vi "main.vi"() -> ()   [LabVIEW 2016]
uses:
  <vilib>/Utility/miscctls.llb/LVMajorAndMinorColorsTypeDef.ctl
panel:
  in  "关闭读取刷新？":bool
  out "项名":string[][](array[string])
  out "下位机消息":T1(array[cluster])
  out "输出数组":T2(array[cluster]) {"Data7" format="%x"; "Data6" format="%x"; "Data5" format="%x"; "Data4" format="%x"; "Data3" format="%x"; "Data2" format="%x"; "Data1" format="%x"; "Data0" format="%x"}
  out "发送配置":T3(array[cluster])
  out "OpenDevice":i32
  out "StartCAN_Success":i32
  out "InitCAN_Success":i32
  out "CloseDevice_Success?":u32
  in  "VCI_INIT_CONFIG":T4={"AccCode"=0, "AccMask"=4294967295, "Reserved"=0, "Filter"=0, "Timing0"=0, "Timing1"=28, "Mode"=0} {"AccCode" format="%x"; "AccMask" format="%x"; "Reserved" format="%x"; "Timing1" format="%x"}
  out "项标识符":string
  in  "选项卡控件":enum32{"通用设置", "实时波形", "数据发送", "历史波形"}(tab)
  in  "远程帧标志：":u8
  in  "上传ID":u32=270 format="%x"
  out "启动日志":string
  in  "输出配置路径":path=path "C:/Users/Azmat/Desktop/canTools_v1.0.0/Confs/Send/发送协议.txt"
  in  "掩码：":u32=4294967295 format="%x"
  in  "校验码：":u32 format="%x"
  in  "波特率：":enum16{"100k", "250k", "500k"}(ring)=enum."250k"
  in  "内存地址":u32=15360 format="%x"
  in  "标定站地址":u32=1 format="%x"
  in  "输入配置路径":path=path "C:/Users/Azmat/Desktop/canTools_v1.0.0/Confs/Receive/接收协议.txt"
  in  "颜色库":u32[](array[colorbox])=[16731714, 16769743, 4390903, 16746746, 4390806, 9603948, 16744793, 4481339, 5898174, 16860, 16766786, 16729344, 4390770, 5963865, 16752520, 15597823, 16775072, 46792, 16730368, 7115393, 10122379, 7465727, 7663, 9306367, 16722686, 11800064, 15663104, 3949056, 16752873, 11121548, 2031753, 12976056]
  in  "标定ID":u32=269 format="%x"
  in  "设备索引号：":u32
  in  "Timing0":u8
  in  "Timing1":u8=28 format="%x"
  out "系统状态":bool
  in  "保存波形":bool
  out "Waveform Chart":dbl[][](graph)
  in  "Chart legend":T5(array[cluster])
  in  "启动":bool
  in  "保存发送表":bool
  in  "搜索发送表":bool
  in  "上传":bool
  in  "下载":bool
  in  "发送表":i32[](listbox) caption="多列列表框"
  in  "打开TDMS":bool
  out "波形图":waveform(dbl)[](graph)
  in  "波形图图例":T6(array[cluster])
  in  "开始":dbl
  in  "结束":dbl
  in  "输入/拖动":bool
  out "波形数组out":dbl[](array[numeric])
  out "接受协议数组":T7(array[cluster])
  out "VCI_CAN_OBJ":T8
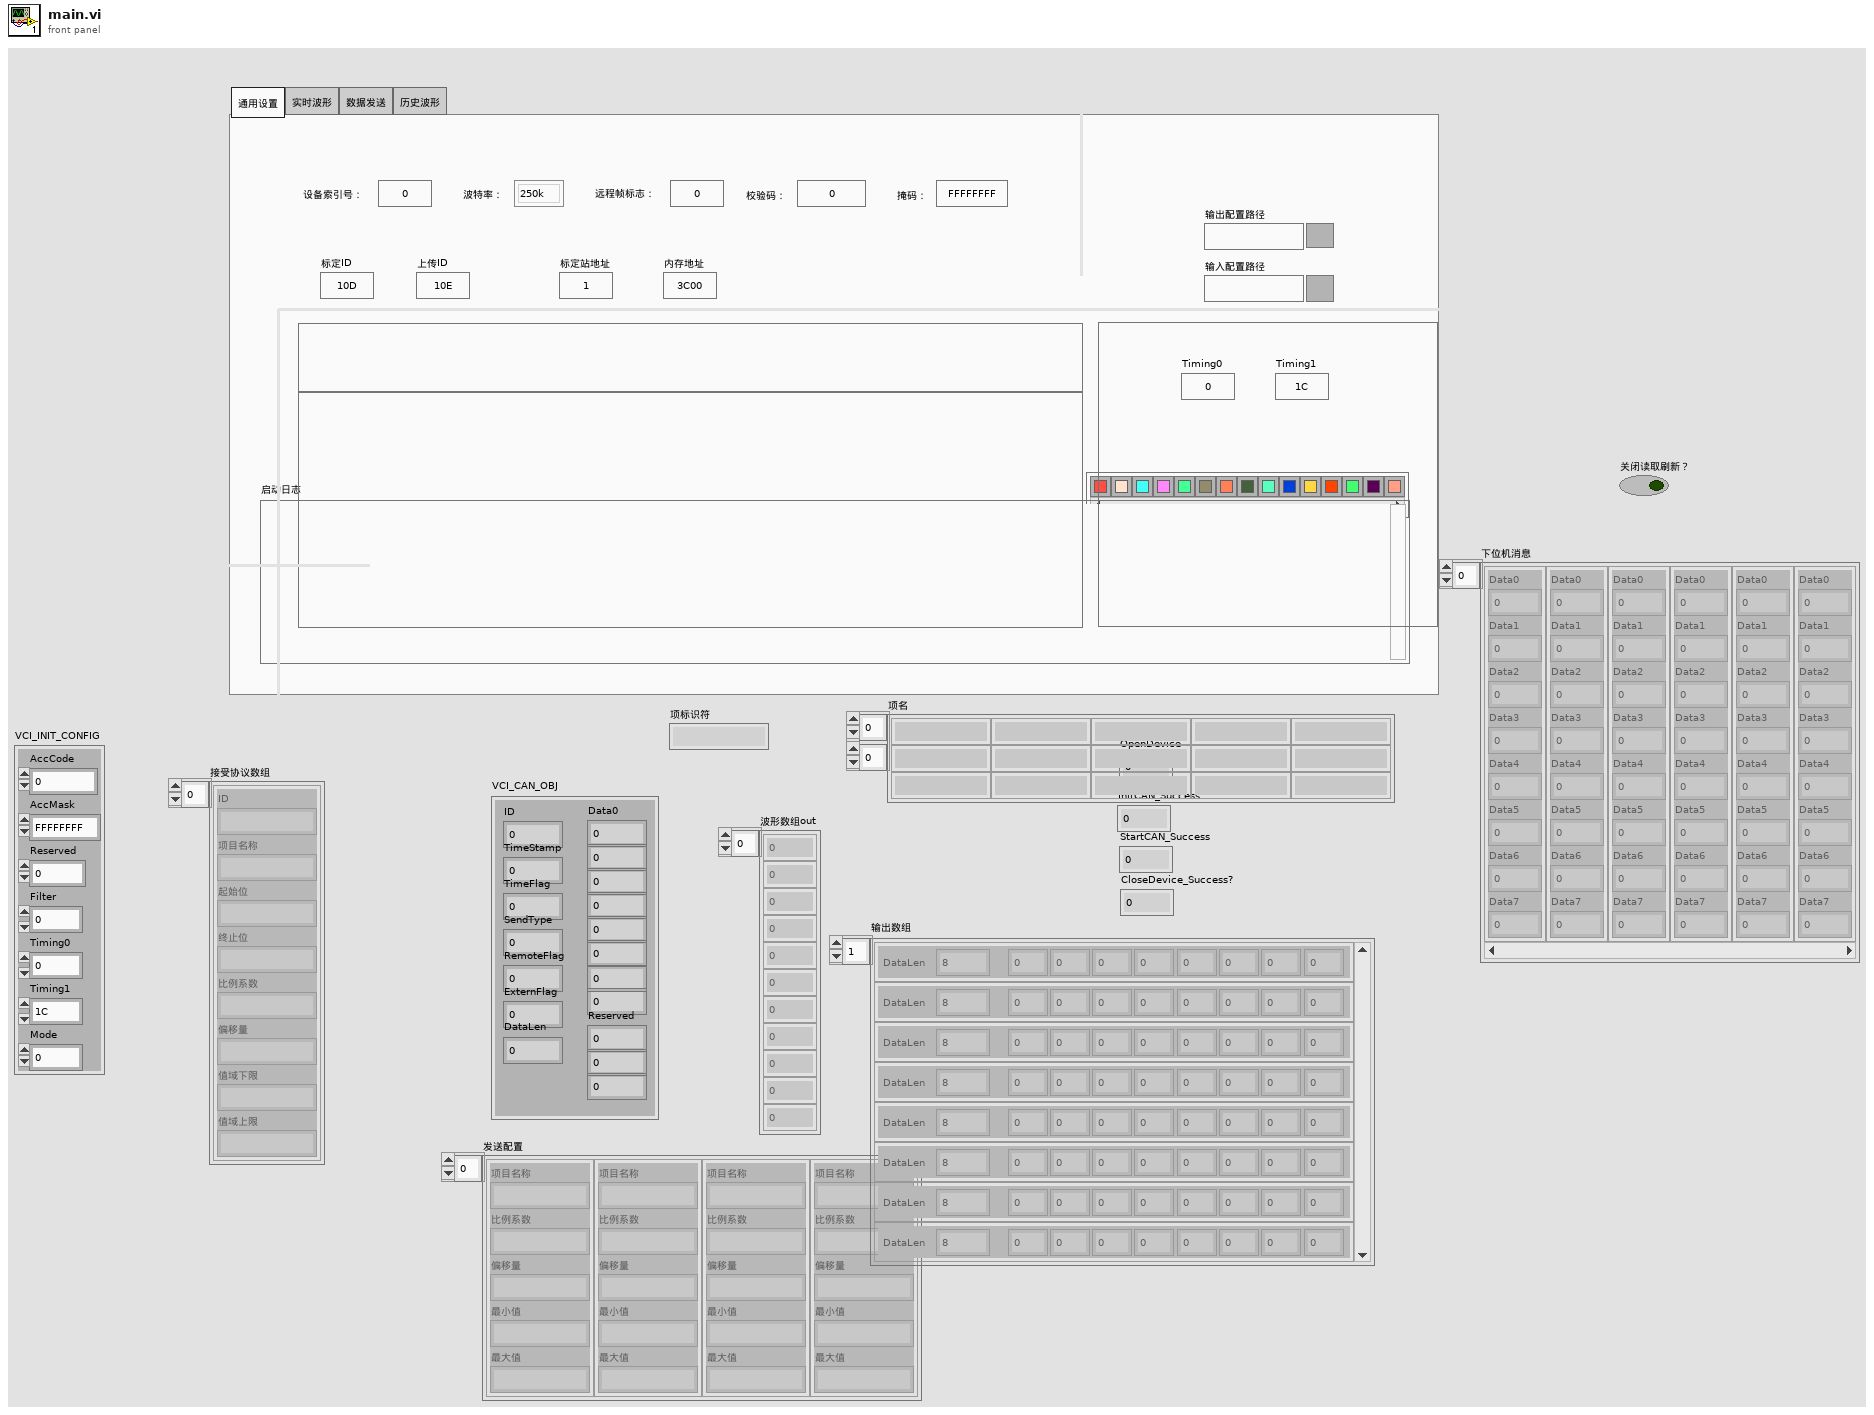
[diagram p1: front panel]
types:
  T1 = cluster{"Data0":u8, "Data1":u8, "Data2":u8, "Data3":u8, "Data4":u8, "Data5":u8, "Data6":u8, "Data7":u8}[]
  T2 = cluster{"Data0":u8, "Data1":u8, "Data2":u8, "Data3":u8, "Data4":u8, "Data5":u8, "Data6":u8, "Data7":u8, "DataLen":u8}[]
  T3 = cluster{"项目名称":string, "比例系数":string, "偏移量":string, "最小值":string, "最大值":string}[]
  T4 = cluster{"AccCode":u32, "AccMask":u32, "Reserved":u32, "Filter":u8, "Timing0":u8, "Timing1":u8, "Mode":u8}
  T5 = cluster{"曲线名称":string, "曲线颜色":u32, "曲线宽度":u16, "当前波形值":dbl, "曲线可见":bool}[]
  T6 = cluster{"曲线名称":string, "曲线颜色":u32, "曲线宽度":u16, "开始":dbl, "曲线可见":bool, "结束":dbl}[]
  T7 = cluster{"ID":string, "项目名称":string, "起始位":string, "终止位":string, "比例系数":string, "偏移量":string, "值域下限":string, "值域上限":string}[]
  T8 = cluster{"ID":u32, "TimeStamp":u32, "TimeFlag":u8, "SendType":i8, "RemoteFlag":u8, "ExternFlag":u8, "DataLen":u8, "Data0":u8, "Data1":u8, "Data2":u8, "Data3":u8, "Data4":u8, "Data5":u8, "Data6":u8, "Data7":u8, "Reserved":u8, u8, u8}
  T9 = cluster{"曲线名称":string, "曲线颜色":u32, "曲线宽度":u16, "当前波形值":dbl, "曲线可见":bool}
  T10 = cluster{"ID":u32, "TimeStamp":u32, "TimeFlag":u8, "SendType":u8, "RemoteFlag":u8, "ExternFlag":u8, "DataLen":u8, "Data0":u8, "data1":u8, "data2":u8, "data3":u8, "data4":u8, "data5":u8, "data6":u8, "data7":u8, "Reserved":u8, u8, u8}
  T11 = enum16{"open", "open or create", "create or replace", "create", "open (read-only)"}
  T12 = cluster{"曲线名称":string, "曲线颜色":u32, "曲线宽度":u16, "开始":dbl, "曲线可见":bool, "结束":dbl}
  T13 = cluster{"data2":u8, "data3":u8, "data4":u8, "data5":u8, "data6":u8, "data7":u8}[]
  T14 = typedef "LVMajorAndMinorColorsTypeDef.ctl" = cluster{"Major Color":u32, "Minor Color":u32}
  T15 = cluster{"曲线名称":string, "曲线颜色":u32, "曲线宽度":u16, "最小值":dbl, "曲线可见":bool, "最大值":dbl}[]
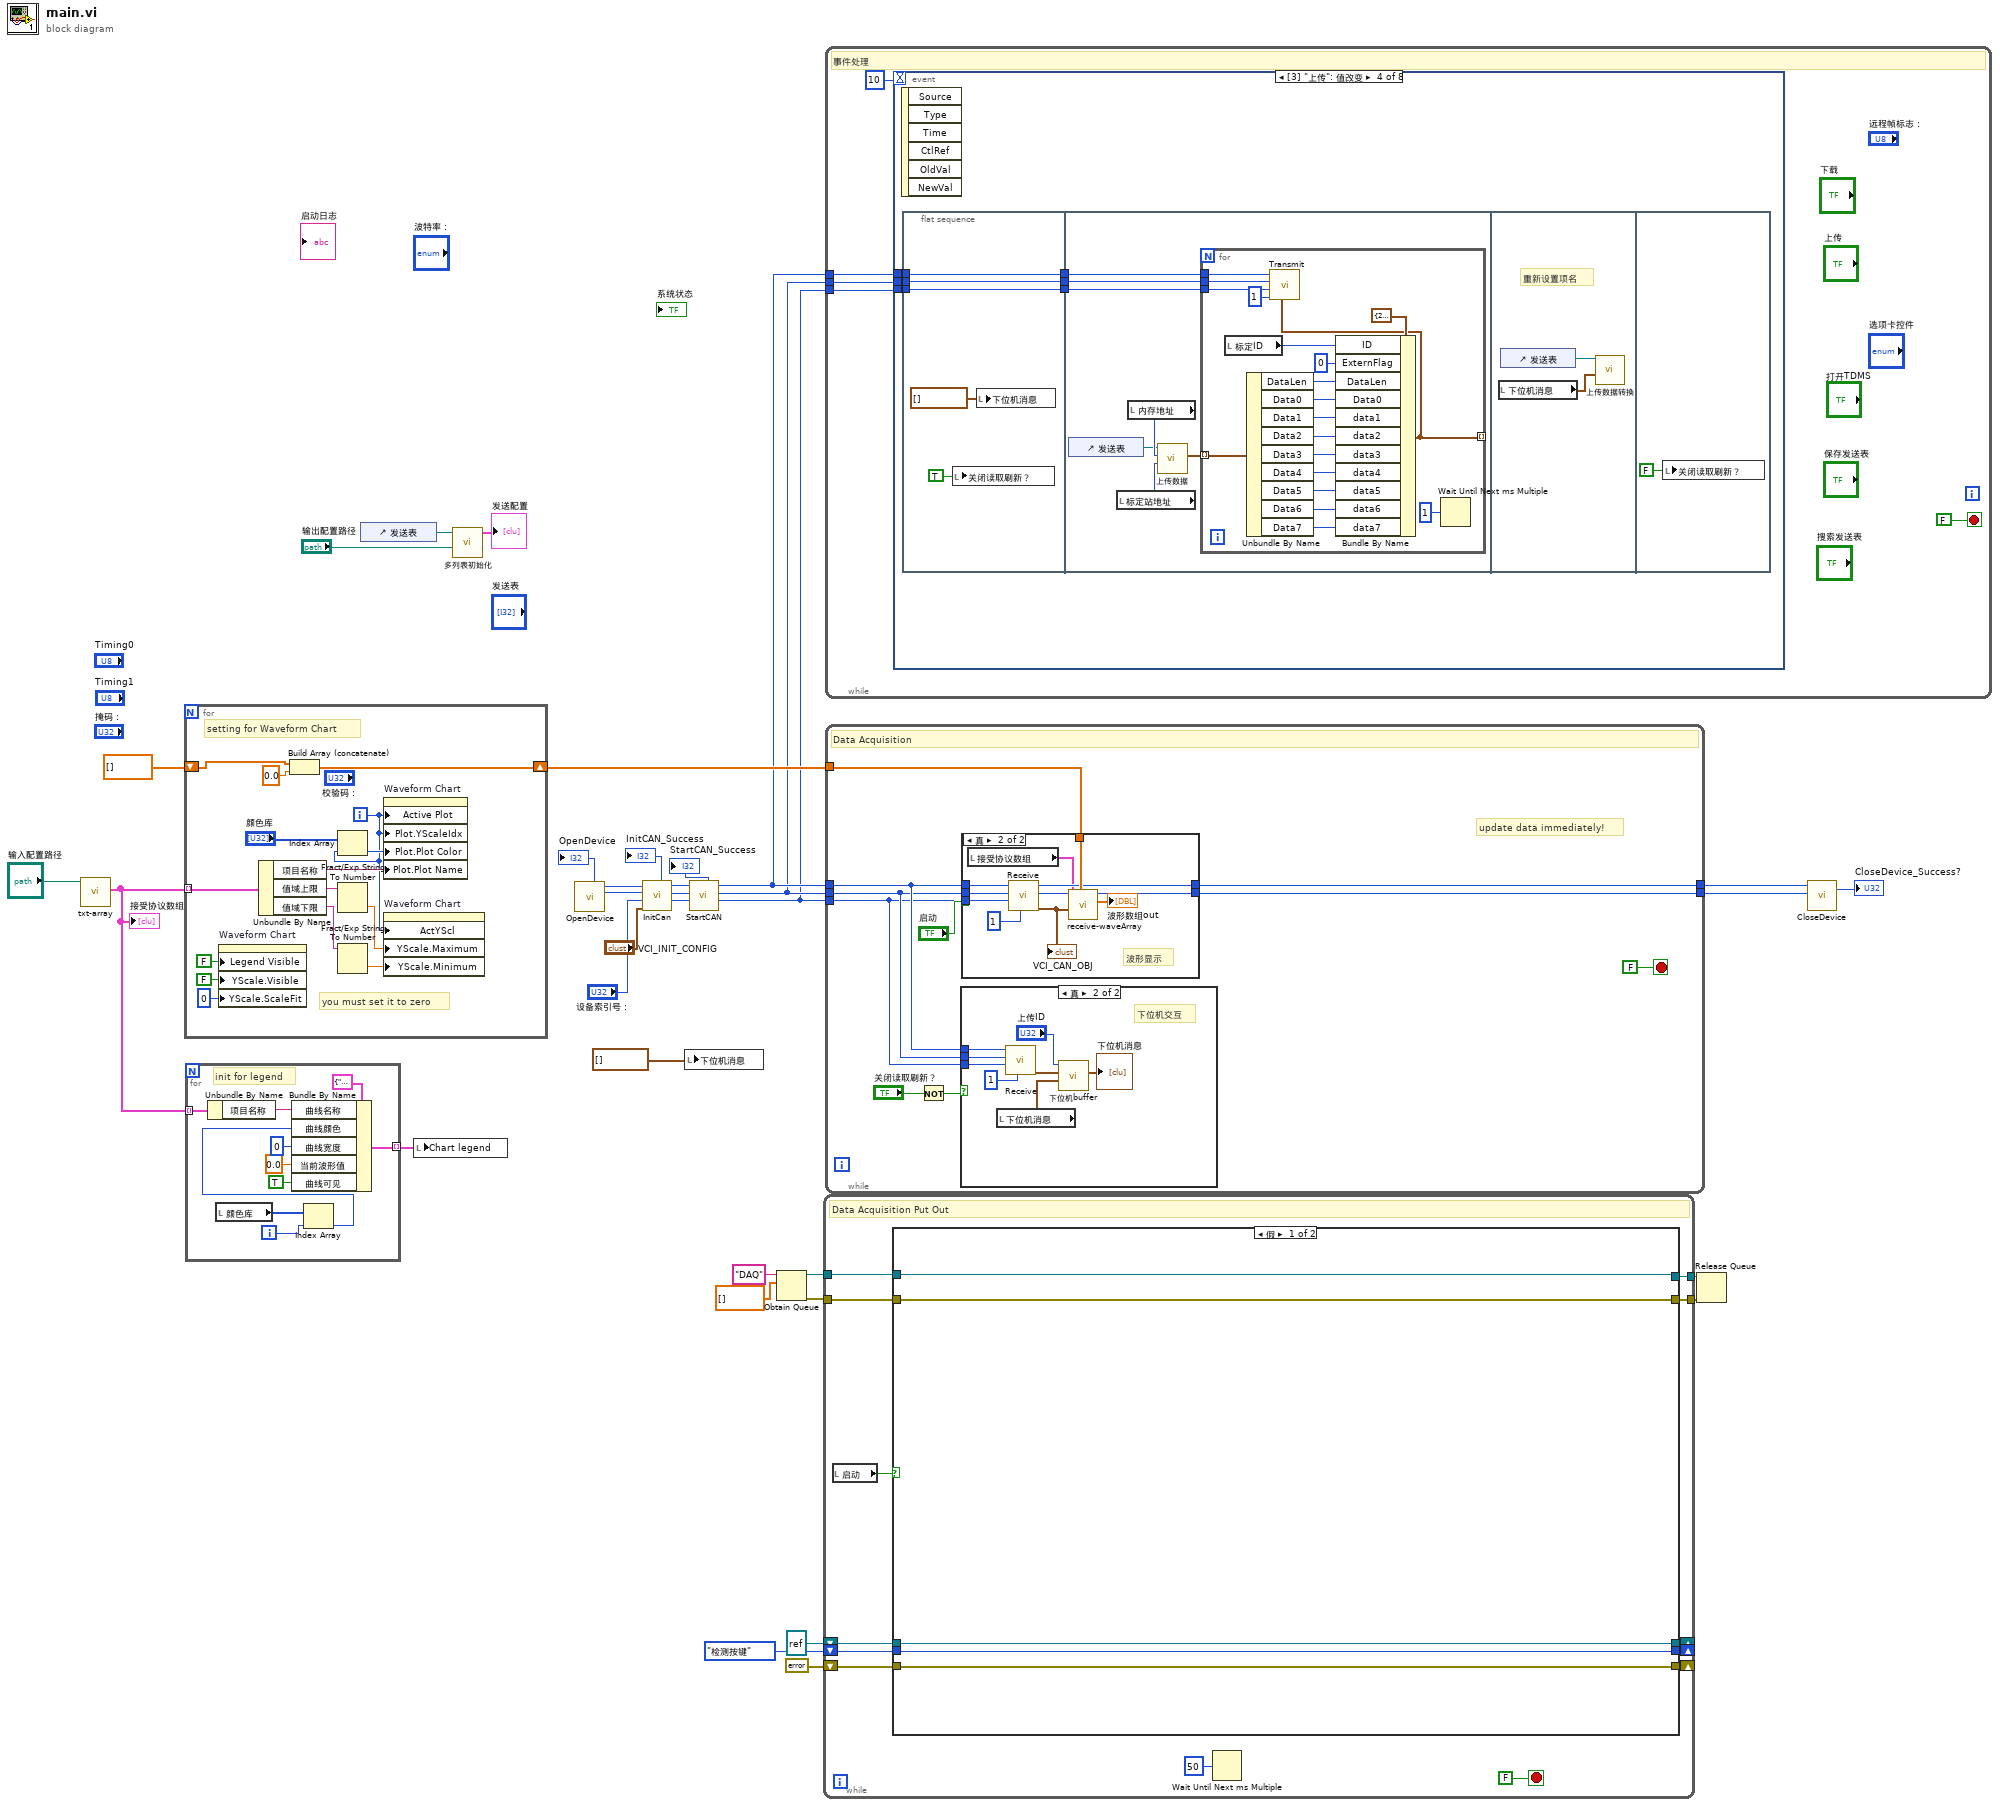
[diagram p0: block diagram]
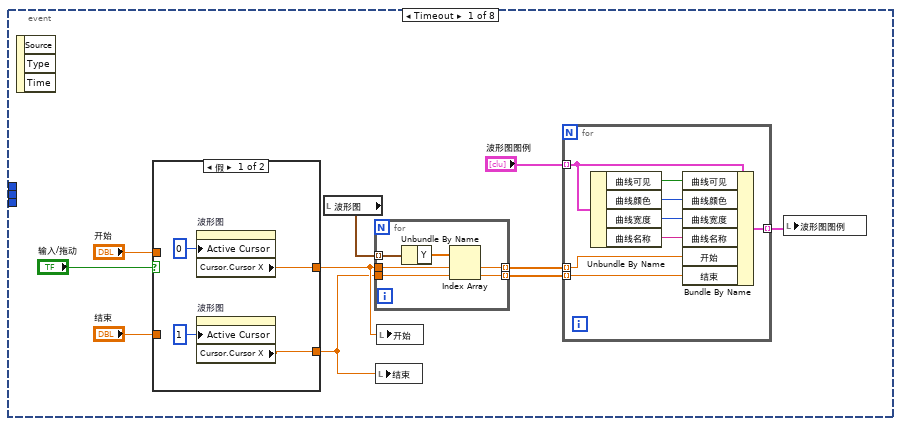
[diagram p2: hidden frame]
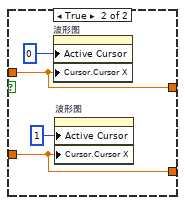
[diagram p3: hidden frame]
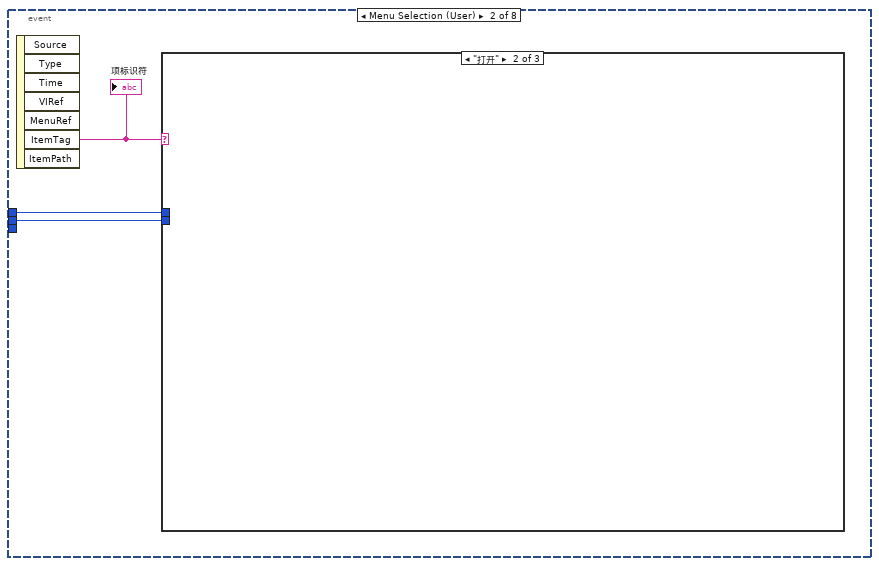
[diagram p4: hidden frame]
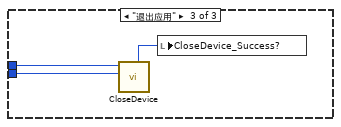
[diagram p6: hidden frame]
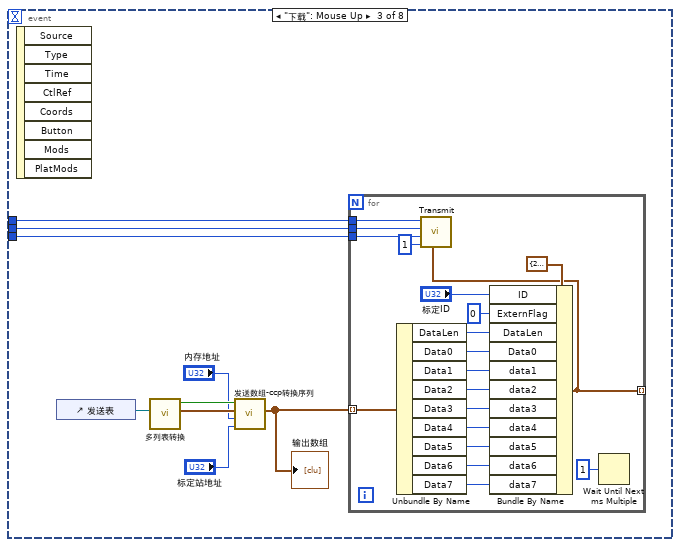
[diagram p7: hidden frame]
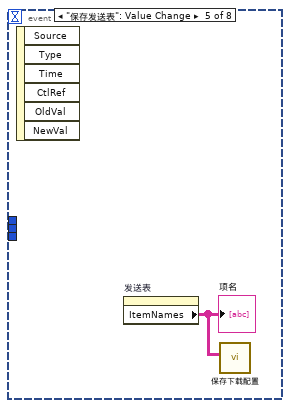
[diagram p8: hidden frame]
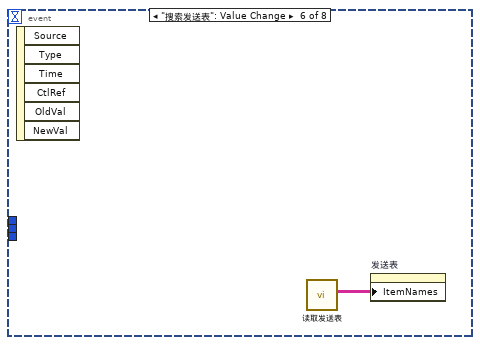
[diagram p9: hidden frame]
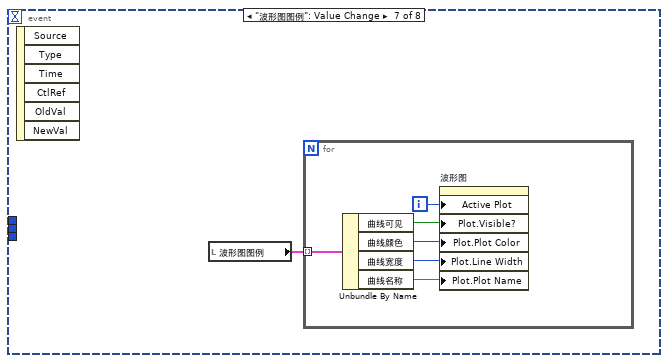
[diagram p10: hidden frame]
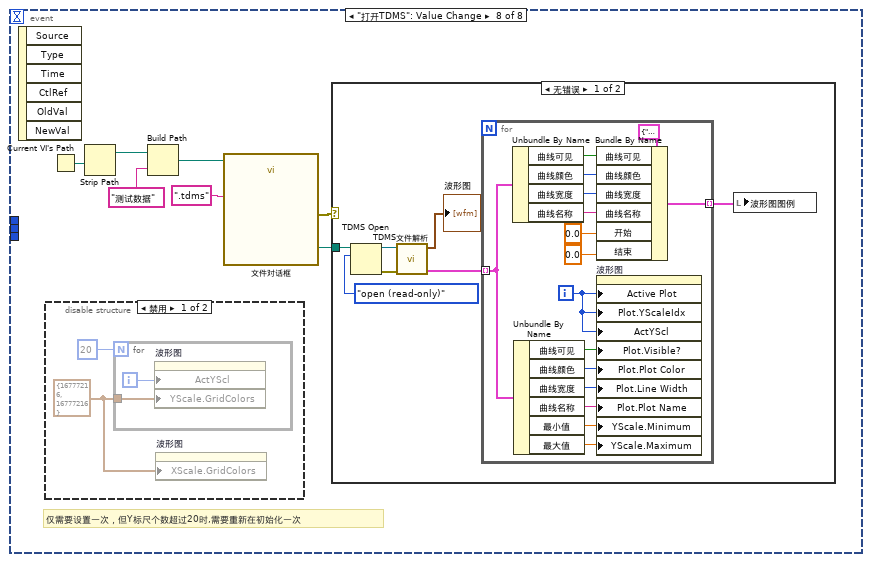
[diagram p11: hidden frame]
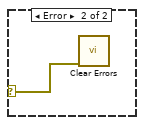
[diagram p12: hidden frame]
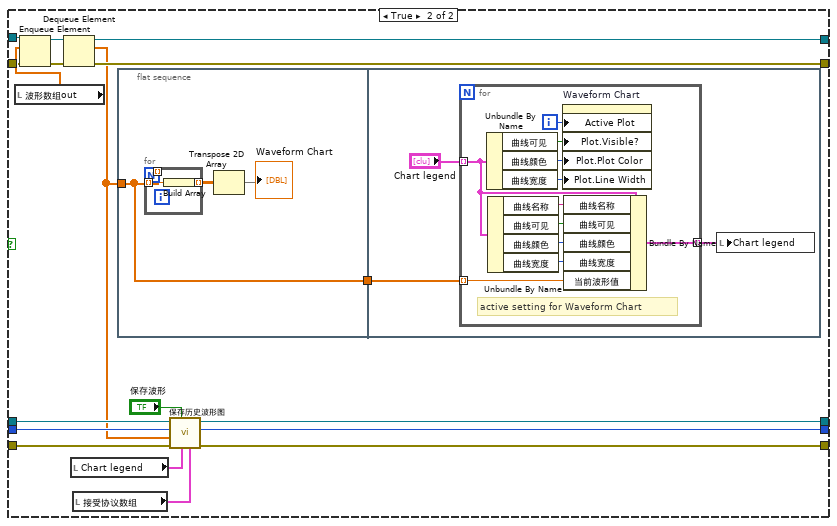
[diagram p14: hidden frame]
diagram:
  n1 = call "txt-array.vi"("file (use dialog)"="输入配置路径") -> ("输出数组"=w23:T7)  [unwired: 9 in]
  "接受协议数组" <- w23
  n2 = for {
    tunnel: w23 -> [w47] mode=indexing
    shift-right: [w36] -> w13
    shift-left: dbl[] [] -> [w35]
    i -> [w41]
    # "you must set it to zero"
    # "setting for Waveform Chart"
    n3 = property on="Waveform Chart" class="WFChart (严格)"("Legend Visible"=FALSE ("Legend:Visible"), "YScale.Visible"=FALSE ("Y Scale.Visible"), "YScale.ScaleFit"=u8 0 ("Y Scale.Scale Fit")) -> ()  [unwired: 2 in, 2 out]
    n4 = Unbundle By Name(w47) -> ("项目名称"=w42:string, "值域上限"=w46:string, "值域下限"=w45:string)
    n5 = Build Array (concatenate)(w35, 0.0) -> (w36:dbl[])
    n6 = Index Array(array="颜色库", index=w41) -> (element=w49:u32)
    n7 = Fract/Exp String To Number(string=w46) -> (number=w44:dbl)  [unwired: 3 in, 1 out]
    n8 = Fract/Exp String To Number(string=w45) -> (number=w43:dbl)  [unwired: 3 in, 1 out]
    n9 = property on="Waveform Chart" class="WFChart (严格)"("Active Plot"=w41, "Plot.YScaleIdx"=w41, "Plot.Plot Color"=w49, "Plot.Plot Name"=w42) -> ()  [unwired: 2 in, 2 out]
    n10 = property on="Waveform Chart" class="WFChart (严格)"("ActYScl"=w41, "YScale.Maximum"=w44, "YScale.Minimum"=w43) -> ()  [unwired: 2 in, 2 out]
  }
  n11 = for {
    tunnel: w23 -> [w59] mode=indexing
    tunnel: [w50] -> w34 mode=indexing
    i -> [w55]
    # "init for legend"
    n12 = Unbundle By Name(w59) -> ("项目名称"=w57:string)
    n13 = local read "颜色库"() -> (w56:u32[])
    n14 = Index Array(array=w56, index=w55) -> (element=w54:u32)
    n15 = Bundle By Name(cluster=T9 {"曲线名称"="", "曲线颜色"=0, "曲线宽度"=0, "当前波形值"=0.0, "曲线可见"=FALSE} ("曲线属性"), "曲线名称"=w57, "曲线颜色"=w54, "曲线宽度"=u16 0, "当前波形值"=0.0, "曲线可见"=TRUE) -> (w50:T9)
  }
  n16 = control-ref of="发送表"() -> (w4:refnum<vi>)
  n17 = local write "Chart legend"(w34) -> ()
  n18 = call "多列表初始化.vi"("配置文件路径"="输出配置路径", "多列列表框"=w4) -> ("发送配置"=→"发送配置":T3)  [unwired: 7 in]
  n19 = call "OpenDevice.vi"() -> ("DevIndex"=w31:u32, "DevType"=w32:u32, "OpenDevice"=→"OpenDevice":i32)  [unwired: 9 out]
  n20 = call "InitCan.vi"("VCI_INIT_CONFIG"="VCI_INIT_CONFIG", "CanIndex_IN"="设备索引号：", "DevIndex_IN"=w31, "DevType_IN"=w32) -> ("CanIndex_OUT"=w26:u32, "DevIndex_OUT"=w27:u32, "DevType_OUT"=w25:u32, "InitCAN_Success?"=→"InitCAN_Success":u32)  [unwired: 4 out]
  n21 = local write "下位机消息"(T1 [] ("输出数组")) -> ()
  n22 = call "StartCAN.vi"("CANIndex"=w26, "DevIndex"=w27, "DevType"=w25) -> ("CANIndex 2"=w9:u32, "DevIndex 2"=w10:u32, "DevType 2"=w11:u32, "StartCAN_Success?"=→"StartCAN_Success":u32)  [unwired: 5 out]
  n23 = Obtain Queue(name (unnamed)="DAQ", element data type=dbl[] []) -> (queue out=w16:refnum<queue>, error out=w18:errorcluster)  [unwired: 3 in, 1 out]
  n24 = while {
    tunnel: w16 -> [w62]
    tunnel: [w70] -> w17
    tunnel: w18 -> [w61]
    tunnel: [w69] -> w19
    shift-right: [w67] -> _
    shift-left: refnum<k34> refnum ("tdms file in") -> [w68]
    shift-right: [w65] -> _
    shift-left: enum16{"检测按键", "设置路径", "保存数据", "关闭TDMS"}."检测按键" -> [w66]
    shift-right: [w63] -> _
    shift-left: errorcluster {"status"=FALSE, "code"=0, "source"=""} ("错误输入") -> [w64]
    stop <- FALSE stop-if-true
    # "Data Acquisition Put Out"
    n25 = local read "启动"() -> (w60:bool)
    n26 = case shown="假" w60 {
      tunnel: [w77 w94] -> w70
      tunnel: [w76 w93] -> w69
      tunnel: w68 -> [w75 w92]
      tunnel: [w75 w91] -> w67
      tunnel: w66 -> [w74 w90]
      tunnel: [w74 w89] -> w65
      tunnel: w64 -> [w73 w88]
      tunnel: [w73 w87] -> w63
      tunnel: w62 -> [w77 w79]
      tunnel: w61 -> [w76 w78]
      frame False {
      }
      frame True {
        n27 = local read "波形数组out"() -> (w82:dbl[])
        n28 = Enqueue Element(queue=w79, element=w82, error in (no error)=w78) -> (queue out=w81:refnum<queue>, error out=w80:errorcluster)  [unwired: 1 in, 1 out]
        n29 = Dequeue Element(queue=w81, error in (no error)=w80) -> (queue out=w94:refnum<queue>, element=w86:dbl[], error out=w93:errorcluster)  [unwired: 1 in, 1 out]
        n30 = local read "Chart legend"() -> (w85:T5)
        n31 = local read "接受协议数组"() -> (w84:T7)
        n32 = flat-sequence {
          tunnel: w86 -> [w96]
          tunnel: [w96] -> w95
          tunnel: w95 -> [w101]
          frame #0 {
            n33 = for {
              tunnel: [w100] -> _ mode=indexing
              tunnel: w96 -> [w100] mode=indexing
              tunnel: [w99] -> w97 mode=indexing
              n34 = Build Array(w100) -> (w99:dbl[])
            }
            n35 = Transpose 2D Array(2D array=w97) -> (transposed array=→"Waveform Chart":dbl[][])
          }
          frame #1 {
            n36 = for {
              tunnel: "Chart legend" -> [w110] mode=indexing
              tunnel: [w106] -> w102 mode=indexing
              tunnel: w101 -> [w105] mode=indexing
              i -> [w112]
              # "active setting for Waveform Chart"
              n37 = Unbundle By Name(w110) -> ("曲线可见"=w114:bool, "曲线颜色"=w113:u32, "曲线宽度"=w111:u16)
              n38 = Unbundle By Name(w110) -> ("曲线名称"=w104:string, "曲线可见"=w109:bool, "曲线颜色"=w108:u32, "曲线宽度"=w107:u16)
              n39 = property on="Waveform Chart" class="WFChart (严格)"("Active Plot"=w112, "Plot.Visible?"=w114, "Plot.Plot Color"=w113, "Plot.Line Width"=w111) -> ()  [unwired: 2 in, 2 out]
              n40 = Bundle By Name(cluster=w110, "曲线名称"=w104, "曲线可见"=w109, "曲线颜色"=w108, "曲线宽度"=w107, "当前波形值"=w105) -> (w106:T9)
            }
            n41 = local write "Chart legend"(w102) -> ()
          }
        }
        n42 = call "保存历史波形图.vi"("接受协议数组"=w84, "Chart legend"=w85, "保存开始"="保存波形", "错误输入"=w88, "队列元素"=w86, "输入"=w90, "tdms file in"=w92) -> ("错误输出"=w87:errorcluster, "输出"=w89:enum16{"检测按键", "设置路径", "保存数据", "关闭TDMS"}, "tdms file out"=w91:refnum<k34>)  [unwired: 2 in]
      }
    }
    n43 = Wait Until Next ms Multiple(millisecond multiple=u32 50) -> ()  [unwired: 1 out]
  }
  n44 = while {
    tunnel: w11 -> [w118]
    tunnel: w10 -> [w117]
    tunnel: w9 -> [w116]
    stop <- FALSE stop-if-true
    # "事件处理"
    n45 = event shown="[3] \"上传\": 值改变" {
      selector: _ -> [_ _ _ _ _ _ _ _]
      dyn-events: _ -> [_ _ _ _ _ _ _ _]
      timeout: 10 -> [_ _ _ _ _ _ _ _]
      tunnel: w118 -> [_ w153 w164 w191 _ _ _ _]
      tunnel: w117 -> [_ w152 w165 w190 _ _ _ _]
      tunnel: w116 -> [_ _ w166 w189 _ _ _ _]
      event Timeout {
        n46 = event-data() -> ()  [unwired: 1 in, 3 out]
        n47 = case shown="假" "输入/拖动" {
          tunnel: "开始" -> [_ w150]
          tunnel: "结束" -> [_ w148]
          tunnel: [w146 w150] -> w121
          tunnel: [w144 w148] -> w120
          frame False {
            n48 = property on="波形图" class="WFGraph (严格)"("Active Cursor"=0 ("游标.游标索引")) -> ("Cursor.Cursor X"=w146:dbl)  [unwired: 2 in, 2 out]
            n49 = property on="波形图" class="WFGraph (严格)"("Active Cursor"=1 ("游标.游标索引")) -> ("Cursor.Cursor X"=w144:dbl)  [unwired: 2 in, 2 out]
          }
          frame True {
            n50 = property on="波形图" class="WFGraph (严格)"("Active Cursor"=0 ("游标.游标索引"), "Cursor.Cursor X"=w150) -> ()  [unwired: 2 in, 2 out]
            n51 = property on="波形图" class="WFGraph (严格)"("Active Cursor"=1 ("游标.游标索引"), "Cursor.Cursor X"=w148) -> ()  [unwired: 2 in, 2 out]
          }
        }
        n52 = local read "波形图"() -> (w126:waveform(dbl)[])
        n53 = for {
          tunnel: w121 -> [w143]
          tunnel: w120 -> [w142]
          tunnel: [w141] -> w124 mode=indexing
          tunnel: [w140] -> w123 mode=indexing
          tunnel: w126 -> [w138] mode=indexing
          n54 = Unbundle By Name(w138) -> ("Y"=w139:dbl[])
          n55 = Index Array(array=w139, index #1=w143, index #2=w142) -> (element #1=w141:dbl, element #2=w140:dbl)
        }
        n56 = local write "结束"(w120) -> ()
        n57 = local write "开始"(w121) -> ()
        n58 = for {
          tunnel: "波形图图例" -> [w137] mode=indexing
          tunnel: w124 -> [w136] mode=indexing
          tunnel: w123 -> [w135] mode=indexing
          tunnel: [w130] -> w122 mode=indexing
          n59 = Unbundle By Name(w137) -> ("曲线可见"=w134:bool, "曲线颜色"=w133:u32, "曲线宽度"=w132:u16, "曲线名称"=w131:string)
          n60 = Bundle By Name(cluster=w137, "曲线可见"=w134, "曲线颜色"=w133, "曲线宽度"=w132, "曲线名称"=w131, "开始"=w136, "结束"=w135) -> (w130:T12)
        }
        n61 = local write "波形图图例"(w122) -> ()
      }
      event Menu Selection (User) {
        n62 = event-data() -> ("ItemTag"=w154:string)  [unwired: 1 in, 6 out]
        "项标识符" <- w154
        n63 = case shown="\"打开\"" w154 {
          tunnel: w153 -> [_ _ w157]
          tunnel: w152 -> [_ _ w156]
          frame "假", Default {
          }
          frame "打开" {
          }
          frame "退出应用" {
            n64 = call "CloseDevice.vi"("DevIndex"=w156, "DevType"=w157) -> ("CloseDevice_Success?"=w155:u32)  [unwired: 9 in]
            n65 = local write "CloseDevice_Success?"(w155) -> ()
          }
        }
      }
      event "下载": Mouse Up {
        n66 = event-data() -> ()  [unwired: 1 in, 8 out]
        n67 = control-ref of="发送表"() -> (w163:refnum<vi>)
        n68 = call "多列表转换.vi"("多列列表框"=w163) -> ("输出数组"=w161:T13, "是否剩余"=w162:bool)  [unwired: 9 in]
        n69 = call "发送数组-ccp转换序列.vi"("标定站地址"="标定站地址", "初始地址"="内存地址", "输入数组"=w161, "是否剩余"=w162) -> ("输出数组"=w160:T2)  [unwired: 7 in]
        "输出数组" <- w160
        n70 = for {
          tunnel: w160 -> [w185] mode=indexing
          tunnel: [w168] -> _ mode=indexing
          tunnel: w166 -> [w171]
          tunnel: w165 -> [w170]
          tunnel: w164 -> [w169]
          n71 = Unbundle By Name(w185) -> ("DataLen"=w175:u8, "Data0"=w176:u8, "Data1"=w177:u8, "Data2"=w178:u8, "Data3"=w179:u8, "Data4"=w180:u8, "Data5"=w181:u8, "Data6"=w182:u8, "Data7"=w183:u8)
          n72 = Bundle By Name(cluster=T10 {"ID"=269, "TimeStamp"=0, "TimeFlag"=0, "SendType"=0, "RemoteFlag"=0, "ExternFlag"=0, "DataLen"=8, "Data0"=1, "data1"=1, "data2"=0, "data3"=1, "data4"=0, "data5"=0, "data6"=0, "data7"=0, "Reserved"=0, 0, 0} ("VCI_CAN_OBJ 2"), "ID"="标定ID", "ExternFlag"=u8 0, "DataLen"=w175, "Data0"=w176, "data1"=w177, "data2"=w178, "data3"=w179, "data4"=w180, "data5"=w181, "data6"=w182, "data7"=w183) -> (w168:T10)
          n73 = call "Transmit.vi"("VCI_CAN_OBJ"=w168, "Len"=u32 1, "CANIndex"=w171, "DevIndex"=w170, "DevType"=w169) -> ()  [unwired: 3 in, 4 out]
          n74 = Wait Until Next ms Multiple(millisecond multiple=u32 1 ("毫秒倍数")) -> ()  [unwired: 1 out]
        }
      }
      event "上传": Value Change {
        n75 = event-data() -> ()  [unwired: 1 in, 6 out]
        n76 = flat-sequence {
          tunnel: w189 -> [w194]
          tunnel: w190 -> [w195]
          tunnel: w191 -> [w196]
          tunnel: [w196] -> w188
          tunnel: [w195] -> w187
          tunnel: [w194] -> w186
          tunnel: w188 -> [w203]
          tunnel: w187 -> [w202]
          tunnel: w186 -> [w201]
          frame #0 {
            n77 = local write "关闭读取刷新？"(TRUE ("关闭读取刷新？")) -> ()
            n78 = local write "下位机消息"(T1 [] ("下位机消息")) -> ()
          }
          frame #1 {
            n79 = control-ref of="发送表"() -> (w198:refnum<vi>)
            n80 = local read "标定站地址"() -> (w199:u32)
            n81 = local read "内存地址"() -> (w200:u32)
            n82 = call "上传数据.vi"("标定站地址"=w199, "初始地址"=w200, "多列列表框"=w198) -> ("输出数组"=w197:T2)  [unwired: 8 in]
            n83 = for {
              tunnel: [w207] -> _ mode=indexing
              tunnel: w201 -> [w210]
              tunnel: w202 -> [w209]
              tunnel: w203 -> [w208]
              tunnel: w197 -> [w204] mode=indexing
              n84 = local read "标定ID"() -> (w205:u32)
              n85 = Unbundle By Name(w204) -> ("DataLen"=w213:u8, "Data0"=w214:u8, "Data1"=w215:u8, "Data2"=w216:u8, "Data3"=w217:u8, "Data4"=w218:u8, "Data5"=w219:u8, "Data6"=w220:u8, "Data7"=w221:u8)
              n86 = Bundle By Name(cluster=T10 {"ID"=269, "TimeStamp"=0, "TimeFlag"=0, "SendType"=0, "RemoteFlag"=0, "ExternFlag"=0, "DataLen"=8, "Data0"=1, "data1"=1, "data2"=0, "data3"=1, "data4"=0, "data5"=0, "data6"=0, "data7"=0, "Reserved"=0, 0, 0} ("VCI_CAN_OBJ 2"), "ID"=w205, "ExternFlag"=u8 0, "DataLen"=w213, "Data0"=w214, "data1"=w215, "data2"=w216, "data3"=w217, "data4"=w218, "data5"=w219, "data6"=w220, "data7"=w221) -> (w207:T10)
              n87 = call "Transmit.vi"("VCI_CAN_OBJ"=w207, "Len"=u32 1, "CANIndex"=w210, "DevIndex"=w209, "DevType"=w208) -> ()  [unwired: 3 in, 4 out]
              n88 = Wait Until Next ms Multiple(millisecond multiple=u32 1 ("毫秒倍数")) -> ()  [unwired: 1 out]
            }
          }
          frame #2 {
            # "重新设置项名"
            n89 = local read "下位机消息"() -> (w224:T1)
            n90 = control-ref of="发送表"() -> (w223:refnum<vi>)
            n91 = call "上传数据转换.vi"("下位机消息"=w224, "多列列表框"=w223) -> ()  [unwired: 10 in]
          }
          frame #3 {
            n92 = local write "关闭读取刷新？"(FALSE ("关闭读取刷新？")) -> ()
          }
        }
      }
      event "保存发送表": Value Change {
        n93 = event-data() -> ()  [unwired: 1 in, 6 out]
        n94 = property on="发送表" class="MCListbox (严格)"() -> ("ItemNames"=w226:string[][])  [unwired: 2 in, 2 out]
        "项名" <- w226
        n95 = call "保存下载配置.vi"("输入数组"=w226) -> ()  [unwired: 11 in]
      }
      event "搜索发送表": Value Change {
        n96 = event-data() -> ()  [unwired: 1 in, 6 out]
        n97 = call "读取发送表.vi"() -> ("输入数组"=w227:string[][])  [unwired: 11 in]
        n98 = property on="发送表" class="MCListbox (严格)"("ItemNames"=w227) -> ()  [unwired: 2 in, 2 out]
      }
      event "波形图图例": Value Change {
        n99 = event-data() -> ()  [unwired: 1 in, 6 out]
        n100 = local read "波形图图例"() -> (w228:T6)
        n101 = for {
          tunnel: w228 -> [w233] mode=indexing
          i -> [w234]
          n102 = Unbundle By Name(w233) -> ("曲线可见"=w232:bool, "曲线颜色"=w231:u32, "曲线宽度"=w230:u16, "曲线名称"=w229:string)
          n103 = property on="波形图" class="WFGraph (严格)"("Active Plot"=w234, "Plot.Visible?"=w232, "Plot.Plot Color"=w231, "Plot.Line Width"=w230, "Plot.Plot Name"=w229) -> ()  [unwired: 2 in, 2 out]
        }
      }
      event "打开TDMS": Value Change {
        # "仅需要设置一次，但Y标尺个数超过20时,需要重新在初始化一次"
        n104 = event-data() -> ()  [unwired: 1 in, 6 out]
        n105 = disable-structure shown="禁用" {
          frame Disabled {
            w266 = T14 {"Major Color"=16777216, "Minor Color"=16777216} ("X标尺.网格颜色")
            n106 = for {
              N: 20 -> [_]
              tunnel: w266 -> [w268]
              i -> [w269]
              n107 = property on="波形图" class="WFGraph (严格)"("ActYScl"=w269, "YScale.GridColors"=w268) -> ()  [unwired: 2 in, 2 out]
            }
            n108 = property on="波形图" class="WFGraph (严格)"("XScale.GridColors"=w266) -> ()  [unwired: 2 in, 2 out]
          }
          frame Enabled {
          }
        }
        n109 = Current VI's Path() -> (path=w236:path)
        n110 = Strip Path(path=w236) -> (stripped path=w239:path)  [unwired: 1 out]
        n111 = Build Path(base path=w239, name or relative path="测试数据") -> (appended path=w241:path)
        n112 = call "文件对话框"("start path"=w241, "pattern label"=".tdms") -> ("selected path"=w238:path, "error out"=w235:errorcluster)  [unwired: 10 in, 2 out]
        n113 = case shown="无错误" w235 {
          selector: w235 -> [_ w265]
          tunnel: w238 -> [w247 _]
          frame No Error {
            n114 = TDMS Open(10:T11."open (read-only)" ("操作(0:open)"), 11:w247) -> (0:w246:errorcluster, 3:w245:refnum<k34>)  [unwired: 5 in]
            n115 = call "TDMS文件解析.vi"("错误输入"=w246, "引用句柄输入"=w245) -> ("历史波形图属性"=w243:T15, "data"=→"波形图":waveform(dbl)[])  [unwired: 7 in]
            n116 = for {
              tunnel: w243 -> [w256] mode=indexing
              tunnel: [w259] -> w242 mode=indexing
              i -> [w249]
              n117 = Unbundle By Name(w256) -> ("曲线可见"=w263:bool, "曲线颜色"=w262:u32, "曲线宽度"=w261:u16, "曲线名称"=w258:string)
              n118 = Unbundle By Name(w256) -> ("曲线可见"=w255:bool, "曲线颜色"=w254:u32, "曲线宽度"=w253:u16, "曲线名称"=w252:string, "最小值"=w251:dbl, "最大值"=w250:dbl)
              n119 = Bundle By Name(cluster=T12 {"曲线名称"="", "曲线颜色"=0, "曲线宽度"=0, "开始"=0.0, "曲线可见"=FALSE, "结束"=0.0} ("曲线属性"), "曲线可见"=w263, "曲线颜色"=w262, "曲线宽度"=w261, "曲线名称"=w258, "开始"=0.0 ("当前波形值 2"), "结束"=0.0 ("当前波形值 2")) -> (w259:T12)
              n120 = property on="波形图" class="WFGraph (严格)"("Active Plot"=w249, "Plot.YScaleIdx"=w249, "ActYScl"=w249, "Plot.Visible?"=w255, "Plot.Plot Color"=w254, "Plot.Line Width"=w253, "Plot.Plot Name"=w252, "YScale.Minimum"=w251, "YScale.Maximum"=w250) -> ()  [unwired: 2 in, 2 out]
            }
            n121 = local write "波形图图例"(w242) -> ()
          }
          frame Error {
            n122 = call <vilib>:"Clear Errors.vi"("error in (no error)"=w265) -> ()  [unwired: 5 in, 2 out]
          }
        }
      }
    }
  }
  n123 = while {
    tunnel: w11 -> [w274]
    tunnel: w10 -> [w273]
    tunnel: w9 -> [w272]
    tunnel: w13 -> [w278]
    tunnel: [w277] -> w22
    tunnel: [w276] -> w21
    stop <- FALSE stop-if-true
    # "update data immediately!"
    # "Data Acquisition"
    n124 = Not(x="关闭读取刷新？") -> (.not. x?=w271:bool)
    n125 = case shown="真" w271 {
      tunnel: w274 -> [_ w287]
      tunnel: w273 -> [_ w286]
      tunnel: w272 -> [_ w285]
      frame False {
      }
      frame True {
        # "下位机交互"
        n126 = local read "下位机消息"() -> (w280:T1)
        n127 = call "Receive.vi"("Len"=u32 1, "CANIndex"=w285, "DevIndex"=w286, "DevType"=w287) -> ("VCI_CAN_OBJ"=w282:T8)  [unwired: 1 in, 6 out]
        n128 = call "下位机buffer.vi"("反馈信息组"=w280, "输入消息"=w282, "上传ID"="上传ID") -> ("输出数组"=→"下位机消息":T1)  [unwired: 8 in]
      }
    }
    n129 = case shown="真" "启动" {
      tunnel: w274 -> [w289 w299]
      tunnel: w273 -> [w288 w298]
      tunnel: w272 -> [_ w297]
      tunnel: w278 -> [_ w296]
      tunnel: [w289 w293] -> w277
      tunnel: [w288 w292] -> w276
      frame False {
      }
      frame True {
        # "波形显示"
        n130 = local read "接受协议数组"() -> (w290:T7)
        n131 = call "Receive.vi"("Len"=u32 1, "CANIndex"=w297, "DevIndex"=w298, "DevType"=w299) -> ("VCI_CAN_OBJ"=w295:T8, "DevIndex 2"=w292:u32, "DevType 2"=w293:u32)  [unwired: 1 in, 4 out]
        "VCI_CAN_OBJ" <- w295
        n132 = call "receive-waveArray.vi"("波形数组in"=w296, "VCI_CAN_OBJ"=w295, "输出数组"=w290) -> ("波形数组out"=→"波形数组out":dbl[])  [unwired: 7 in]
      }
    }
  }
  n133 = Release Queue(queue=w17, error in (no error)=w19) -> ()  [unwired: 1 in, 3 out]
  n134 = call "CloseDevice.vi"("DevIndex"=w21, "DevType"=w22) -> ("CloseDevice_Success?"=→"CloseDevice_Success?":u32)  [unwired: 9 in]
